vi "asset.attach_dataset_free.vi"(8 "error in":errorcluster, 11 "AssetAttachDatasetStaging in":refnum<class "AssetAttachDatasetStaging.lvclass">) -> (0 "error out":errorcluster, 3 "AssetAttachDatasetStaging out":refnum<class "AssetAttachDatasetStaging.lvclass">)   [LabVIEW 2020, in "AssetAttachDatasetStaging.lvclass"]
doc: "Releases the handle and its associated resources."
uses:
  AssetAttachDatasetStaging.lvclass
  AssetAttachDatasetStaging.lvclass/AssetAttachDatasetStaging.ctl
  client.lvlib
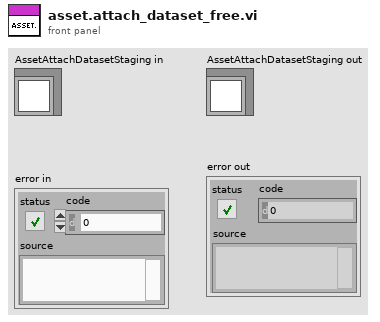
[diagram p1: front panel]
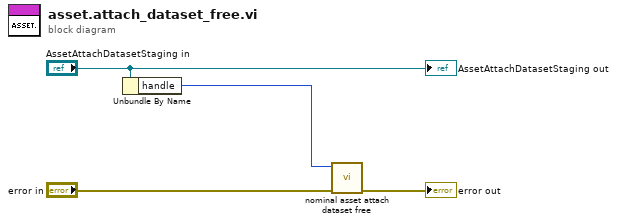
[diagram p0: block diagram]
diagram:
  n1 = Unbundle By Name("AssetAttachDatasetStaging in") -> ("handle"=w2:i32)
  n2 = call "nominal asset attach dataset free.vi"("error in (no error)"="error in", "staging"=w2) -> ("error out"=→"error out":errorcluster)  [unwired: 8 in, 1 out]
  "AssetAttachDatasetStaging out" <- "AssetAttachDatasetStaging in"
